vi "Auto-Refresh Read.vi"(8 "error in (no error)":errorcluster, 11 "DriverMasterSync in":refnum<class "DriverMasterSync.lvclass">) -> (0 "error out":errorcluster, 1 "Control Data":T1, 2 "1 Sample":T2, 3 "DriverMasterSync out":refnum<class "DriverMasterSync.lvclass">)   [LabVIEW 2014, in "DriverMasterSync.lvlib" / "DriverMasterSync.lvclass"]
uses:
  DriverMasterSync.lvclass
  APIs/Data Queue/Acquisition Data 1 Sample Cluster.ctl
  APIs/Data Queue/Control Data Cluster.ctl
  DriverMasterSync.lvclass/DriverMasterSync.ctl
  APIs/Data Queue/WINFAS 2 Data Queue.lvlib
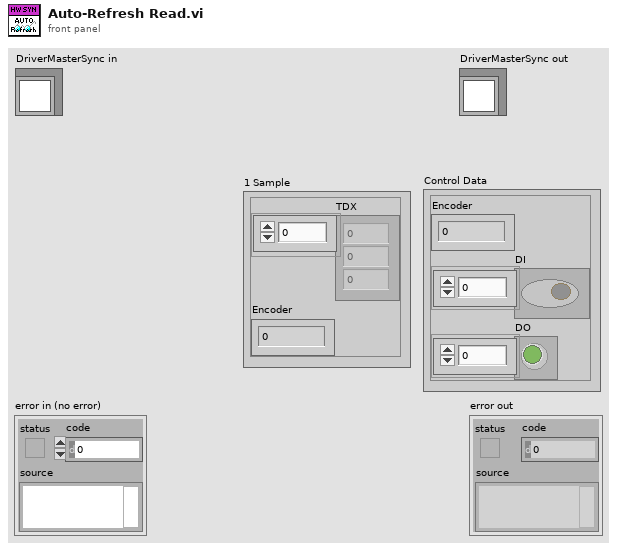
[diagram p1: front panel]
types:
  T1 = typedef "WINFAS 2 Data Queue.lvlib/Control Data Cluster.ctl" = cluster{"Encoder":sgl, "DI":bool[], "DO":bool[]}
  T2 = typedef "WINFAS 2 Data Queue.lvlib/Acquisition Data 1 Sample Cluster.ctl" = cluster{"TDX":sgl[], "Encoder":sgl}
  T3 = typedef "WINFAS 2 Data Queue.lvlib/Acquisition Data Cluster.ctl" = T2[]
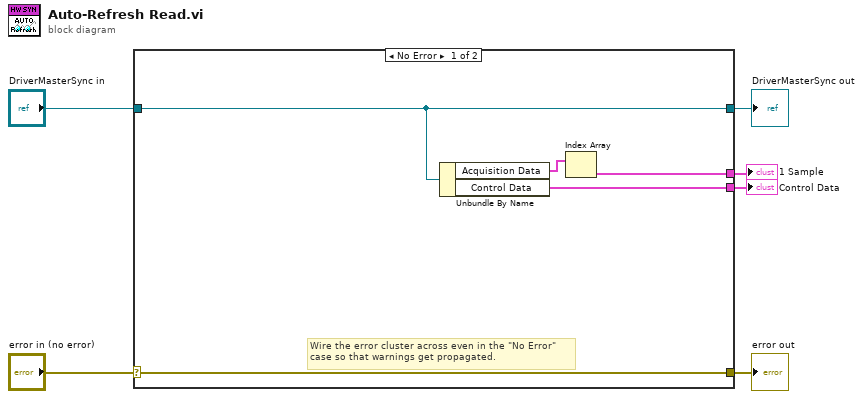
[diagram p0: block diagram]
diagram:
  n1 = case shown="No Error" "error in (no error)" {
    selector: "error in (no error)" -> [w11 w13]
    tunnel: [w11 w13] -> w5
    tunnel: [w10 w12] -> w3
    tunnel: "DriverMasterSync in" -> [w10 w12]
    tunnel: [w9 _] -> w1
    tunnel: [w7 _] -> w2
    frame No Error {
      # "Wire the error cluster across even in the \"No Error\"\ncase so that warnings get propagated."
      n2 = Unbundle By Name(w10) -> ("Acquisition Data"=w8:T3, "Control Data"=w9:T1)
      n3 = Index Array(array=w8) -> (element=w7:T2)  [unwired: 1 in]
    }
    frame Error {
    }
  }
  "error out" <- w5
  "DriverMasterSync out" <- w3
  "1 Sample" <- w2
  "Control Data" <- w1
